vi "Shutdown.vi"(8 "error in (no error)":errorcluster, 9 "timeout in ms (-1)":i32=-1, 11 "TCP_Server in":refnum<class "TCP_Server.lvclass">) -> (0 "error out":errorcluster, 3 "TCP_Server out":refnum<class "TCP_Server.lvclass">)   [LabVIEW 2013, in "TCP_Server.lvclass"]
uses:
  TCP_Server.lvclass
  TCP_Server.lvclass/TCP_Server.ctl
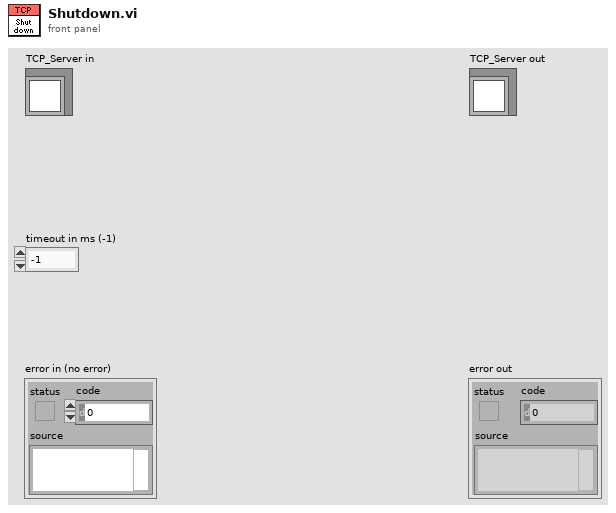
[diagram p1: front panel]
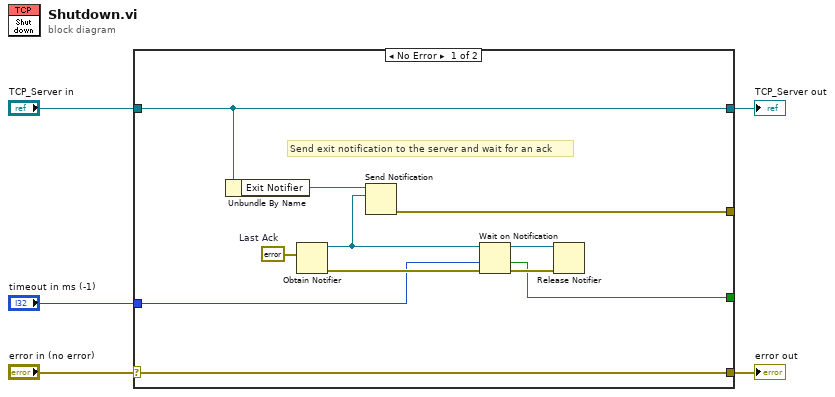
[diagram p0: block diagram]
diagram:
  n1 = case shown="No Error" "error in (no error)" {
    selector: "error in (no error)" -> [w16 w18]
    tunnel: [w16 w18] -> w4
    tunnel: [w15 w17] -> w2
    tunnel: "TCP_Server in" -> [w15 w17]
    tunnel: "timeout in ms (-1)" -> [w10 _]
    tunnel: [w7 _] -> _
    tunnel: [w6 _] -> _
    frame No Error {
      w13 = errorcluster {"status"=FALSE, "code"=0, "source"=""}  # Last Ack
      # "Send exit notification to the server and wait for an ack"
      n2 = Unbundle By Name(w15) -> ("Exit Notifier"=w14:refnum<notifier>)
      n3 = Obtain Notifier(notification data type=w13) -> (notifier out=w12:refnum<notifier>, error out=w11:errorcluster)  [unwired: 3 in, 1 out]
      n4 = Send Notification(notification=w12, notifier=w14) -> (error out=w7:errorcluster)  [unwired: 1 in, 1 out]
      n5 = Wait on Notification(notifier=w12, timeout in ms (-1)=w10, error in (no error)=w11) -> (notifier out=w9:refnum<notifier>, timed out?=w6:bool, error out=w8:errorcluster)  [unwired: 1 in, 1 out]
      n6 = Release Notifier(notifier=w9, error in (no error)=w8) -> ()  [unwired: 1 in, 3 out]
    }
    frame Error {
    }
  }
  "error out" <- w4
  "TCP_Server out" <- w2
